vi "Registry Test Launcher.vi"() -> ()   [LabVIEW 2014]
uses:
  Registry/NameRegistry.lvclass
  Delimiter/Delimiter.lvclass
  RandomStringGenerator/RandomStringGenerator.lvclass
  UniquenessCriteria/UniquenessCriteria.lvclass
  NameIncrementAlgorithm/StringIncrement.lvclass
  Registry/RegistryConfiguration.ctl
  UniqueNameClass/UniqueName.lvclass
  StringIncrement.Alphabetical/StringIncrement.Alphabetical.lvclass
  UniquenessCriteria/Criteria.ctl
panel:
  in  "Criteria":T1
  out "All Nodes":string[](array[string])
  out "objects remaining":i32
  out "error out":errorcluster
  out "Dependencies removed":string[](array[string])
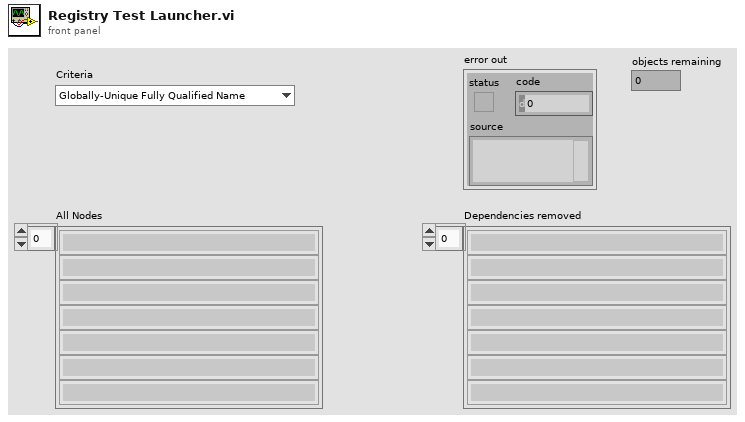
[diagram p1: front panel]
types:
  T1 = typedef "UniquenessCriteria.lvclass/Criteria.ctl" = enum16{"Globally-Unique Fully Qualified Name", "Globally-Unique Name"}
  T2 = typedef "UniqueName.lvlib/NameRegistry.lvclass/RegistryConfiguration.ctl" = cluster{"Delimiter":refnum<class "Delimiter.lvclass">, "RandomStringGenerator":refnum<class "RandomStringGenerator.lvclass">, "UniquenessCriteria":refnum<class "UniquenessCriteria.lvclass">, "StringIncrement":refnum<class "StringIncrement.lvclass">}
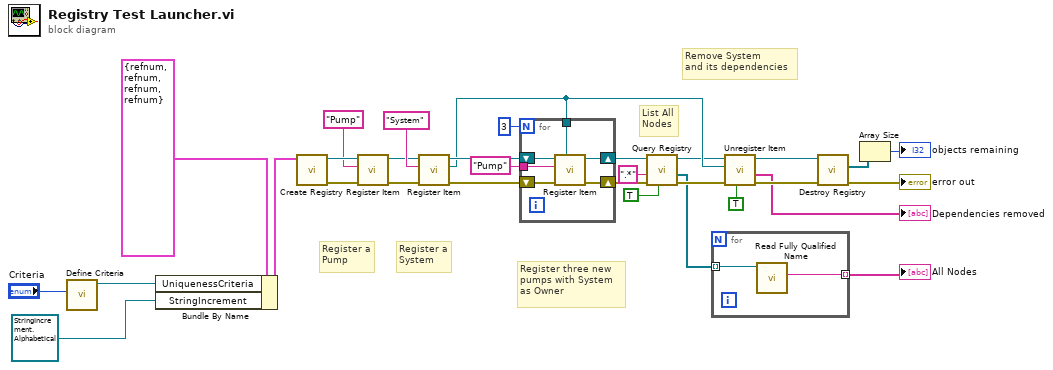
[diagram p0: block diagram]
diagram:
  # "Remove System\nand its dependencies"
  # "List All\nNodes"
  # "Register three new\npumps with System\nas Owner"
  # "Register a\nSystem"
  # "Register a\nPump"
  n1 = call "Define Criteria.vi"("Criteria"="Criteria") -> ("UniquenessCriteria out"=w16:refnum<class "UniquenessCriteria.lvclass">)  [unwired: 10 in]
  n2 = Bundle By Name(cluster=T2 {"Delimiter"=refnum, "RandomStringGenerator"=refnum, "UniquenessCriteria"=refnum, "StringIncrement"=refnum} ("Registry Configuration"), "UniquenessCriteria"=w16, "StringIncrement"=refnum<class "StringIncrement.Alphabetical.lvclass"> refnum ("StringIncrement.Alphabetical.lvclass")) -> (w17:T2)
  n3 = call "Create Registry.vi"("Registry Configuration"=w17) -> ("error out"=w12:errorcluster, "Registry"=w13:refnum<data-value>)  [unwired: 9 in]
  n4 = call "Register Item.vi"("error in (no error)"=w12, "New Object Name"="Pump", "Registry in"=w13) -> ("error out"=w14:errorcluster, "Registry"=w15:refnum<data-value>)  [unwired: 6 in, 1 out]
  n5 = call "Register Item.vi"("error in (no error)"=w14, "New Object Name"="System", "Registry in"=w15) -> ("error out"=w29:errorcluster, "New Node"=w20:refnum<class "UniqueName.lvclass">, "Registry"=w30:refnum<data-value>)  [unwired: 6 in]
  n6 = for {
    N: 3 -> [_]
    shift-right: [w36] -> w10
    shift-left: w30 -> [w37]
    shift-right: [w34] -> w8
    shift-left: w29 -> [w35]
    tunnel: "Pump" ("New Object Name") -> [w33]
    tunnel: w20 -> [w32]
    n7 = call "Register Item.vi"("Owner"=w32, "error in (no error)"=w35, "New Object Name"=w33, "Registry in"=w37) -> ("error out"=w34:errorcluster, "Registry"=w36:refnum<data-value>)  [unwired: 5 in, 1 out]
  }
  n8 = call "Query Registry.vi"("use Regex? (F)"=TRUE, "error in (no error)"=w8, "Search string"=".*", "Registry in"=w10) -> ("error out"=w7:errorcluster, "Nodes"=w4:refnum<class "UniqueName.lvclass">[], "Registry"=w9:refnum<data-value>)  [unwired: 3 in, 2 out]
  n9 = for {
    tunnel: w4 -> [w39] mode=indexing
    tunnel: [w38] -> w3 mode=indexing
    n10 = call "Read Fully Qualified Name.vi"("UniqueName in"=w39) -> ("Fully Qualified Name"=w38:string)  [unwired: 9 in, 1 out]
  }
  "All Nodes" <- w3
  n11 = call "Unregister Item.vi"("Remove Dependencies?"=TRUE, "error in (no error)"=w7, "Node"=w20, "Registry in"=w9) -> ("error out"=w27:errorcluster, "Dependencies removed"=→"Dependencies removed":string[], "Registry"=w31:refnum<data-value>)  [unwired: 4 in, 1 out]
  n12 = call "Destroy Registry.vi"("error in (no error)"=w27, "Registry in"=w31) -> ("error out"=→"error out":errorcluster, "Remaining Nodes"=w2:refnum<class "UniqueName.lvclass">[])  [unwired: 8 in]
  n13 = Array Size(array=w2) -> (size(s)=→"objects remaining":i32)
